vi "MatrixSwitch.vi"(8 "error in (no error)":errorcluster, 10 "Action":T1(ring), 11 "Pickering in":refnum<class "Pickering.lvclass">) -> (0 "error out":errorcluster, 2 "Continue?":bool, 3 "Pickering out":refnum<class "Pickering.lvclass">)   [LabVIEW 2013, in "Pickering.lvclass"]
uses:
  Pickering.lvclass
  InstrumentSetup.vi
  InstrControl.lvclass
panel:
  out "Display Matrix":bool[][](array[boolean])
  # "Pickering Matrix Settings"
  # "X1"
  # "X2"
  # "X3"
  # "X4"
  # "X5"
  # "X6"
  # "X7"
  # "X8"
  # "X9"
  # "X10"
  # "X11"
  # "X12"
  # "Y1"
  # "Y2"
  # "Y3"
  # "Y4"
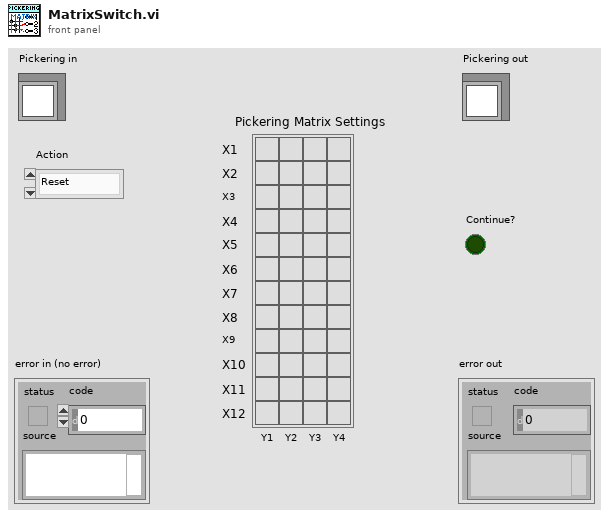
[diagram p1: front panel]
types:
  T1 = enum16{"Reset", "Ground", "Striptest SMU", "Striptest LCR", "IV", "CV", "Interstrip Cap", "Interstrip Res"}
  T2 = cluster{"Matrix address":string, "Mux1 address":string, "Mux2 address":string, "Matrix used?":bool, "Pickering":refnum<class "Pickering.lvclass">, "Matrix X Channels":cluster{"Bias Supply / SMU LO":i32, "Bias Supply / SMU HI":i32, "CV Box LO":i32, "CV Box HI":i32, "CV Box LO IN":i32, "CV Box HI IN":i32, "Volt meter LO":i32, "Volt meter HI":i32, "Mux1 C1":i32, "Mux1 C2":i32, "Mux2 C1":i32, "Mux2 C2":i32}}
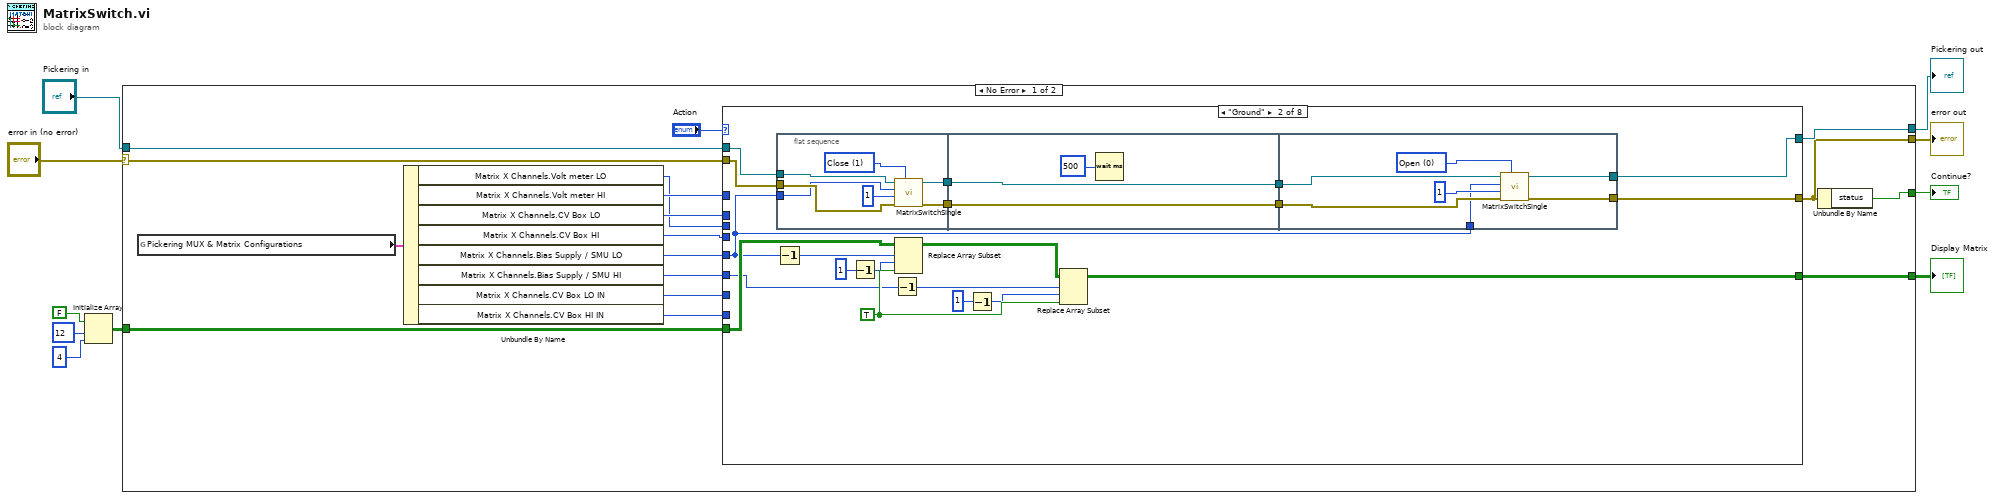
[diagram p0: block diagram]
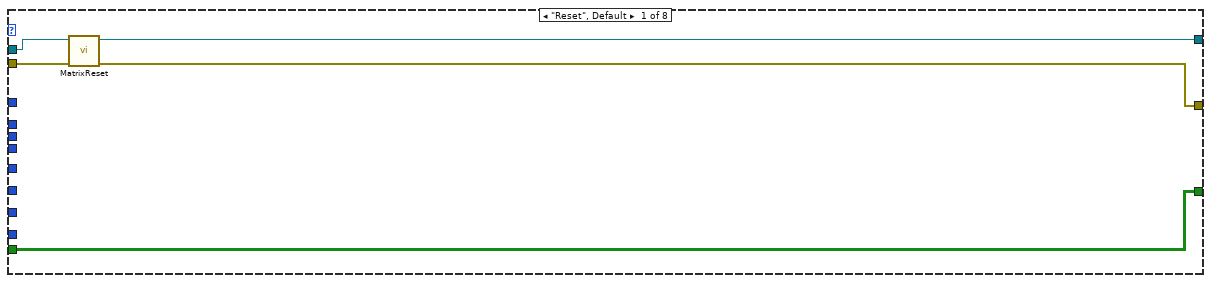
[diagram p2: hidden frame]
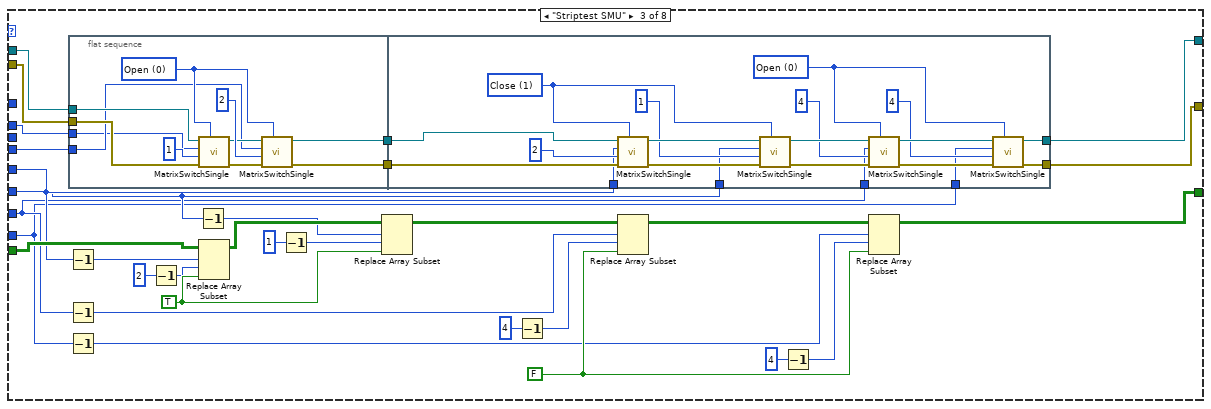
[diagram p3: hidden frame]
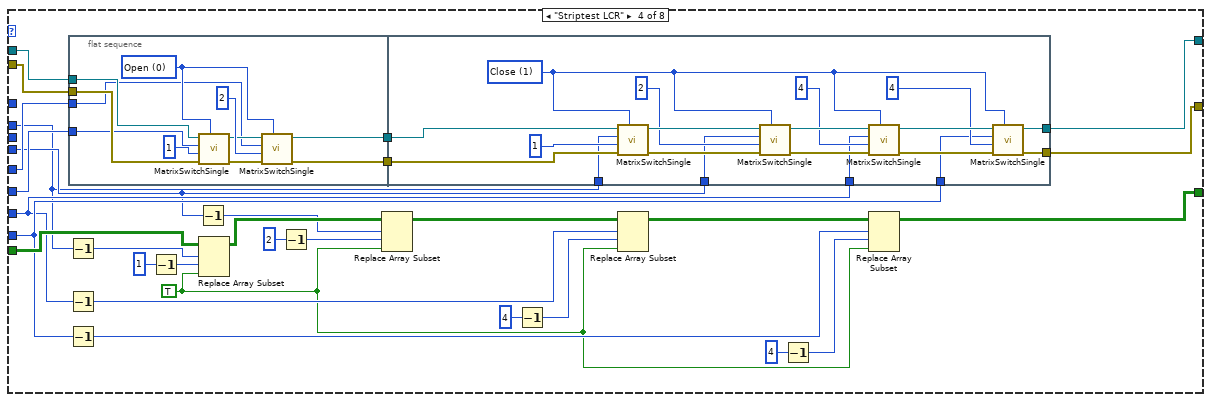
[diagram p4: hidden frame]
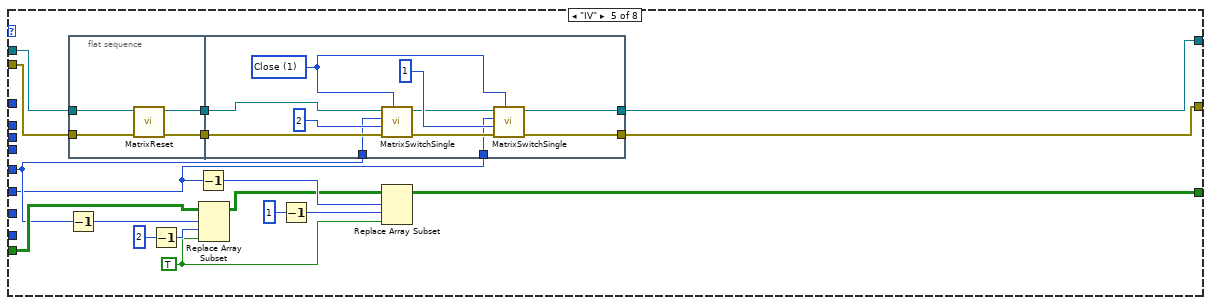
[diagram p5: hidden frame]
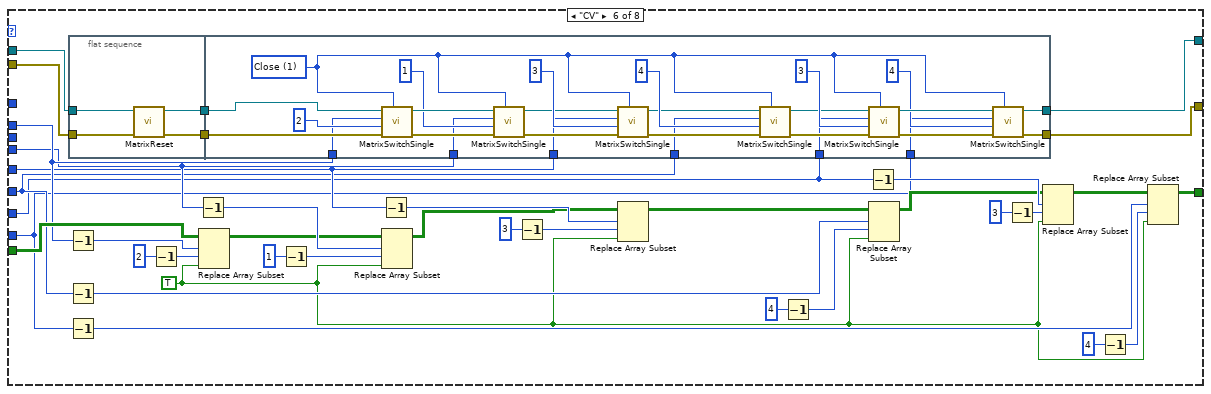
[diagram p6: hidden frame]
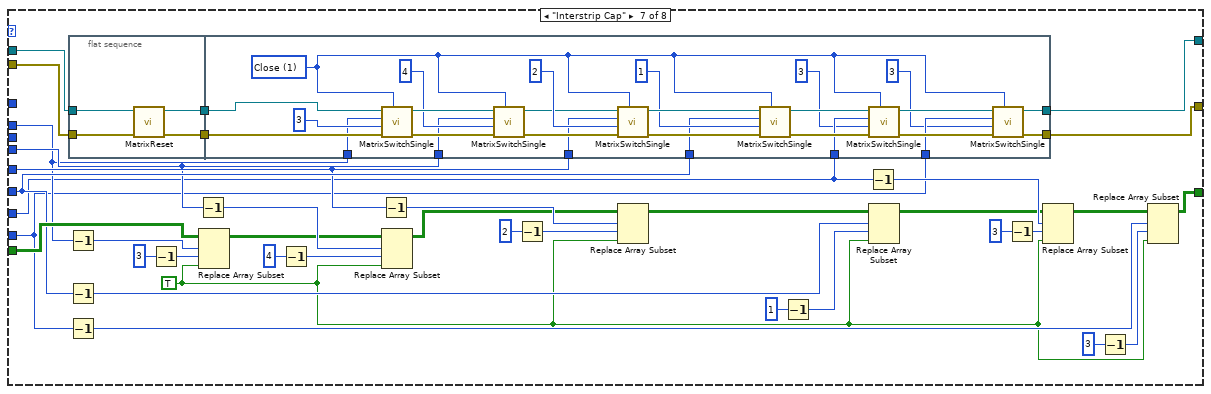
[diagram p7: hidden frame]
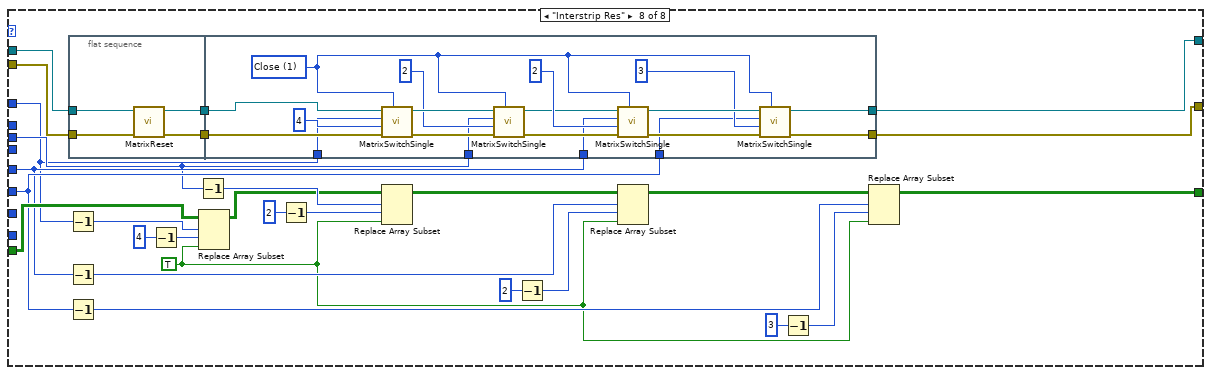
[diagram p8: hidden frame]
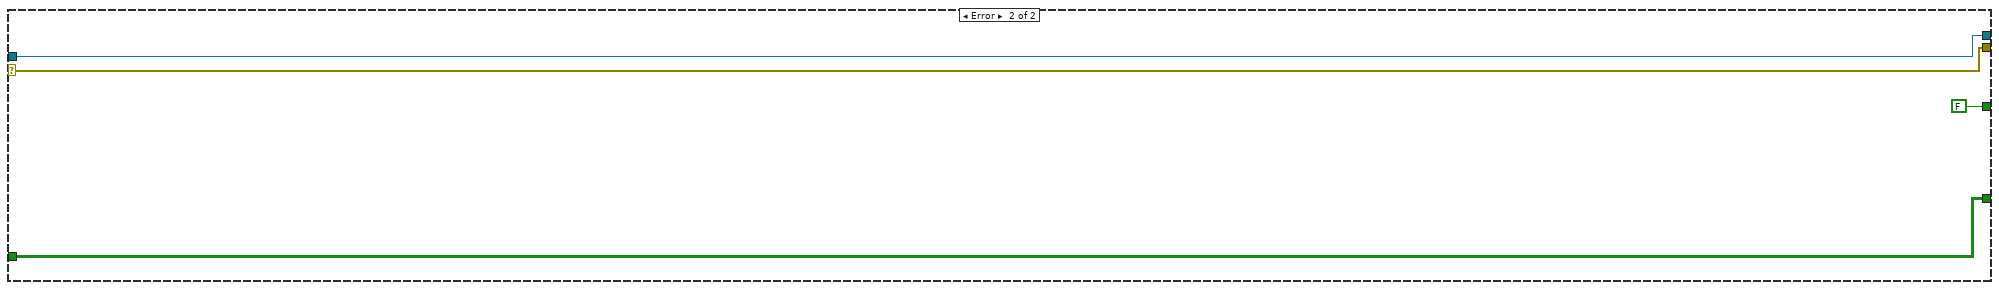
[diagram p9: hidden frame]
diagram:
  n1 = Initialize Array(FALSE, 12, 4) -> (w5:bool[][])
  n2 = case shown="No Error" "error in (no error)" {
    selector: "error in (no error)" -> [w21 w417]
    tunnel: [w24 w417] -> w2
    tunnel: [w25 w416] -> w1
    tunnel: "Pickering in" -> [w22 w416]
    tunnel: [w23 FALSE] -> w4
    tunnel: w5 -> [w27 w414]
    tunnel: [w26 w414] -> w3
    frame No Error {
      n3 = global read "InstrumentSetup.vi" "Pickering MUX & Matrix Configurations"() -> (w20:T2)
      n4 = Unbundle By Name(w20) -> ("Matrix X Channels.Volt meter LO"=w14:i32, "Matrix X Channels.Volt meter HI"=w15:i32, "Matrix X Channels.CV Box LO"=w19:i32, "Matrix X Channels.CV Box HI"=w18:i32, "Matrix X Channels.Bias Supply / SMU LO"=w12:i32, "Matrix X Channels.Bias Supply / SMU HI"=w13:i32, "Matrix X Channels.CV Box LO IN"=w17:i32, "Matrix X Channels.CV Box HI IN"=w16:i32)
      n5 = case shown="\"Ground\"" "Action" {
        tunnel: w27 -> [w32 w37 w87 w150 w200 w237 w317 w375]
        tunnel: [w32 w35 w86 w149 w201 w238 w294 w376] -> w26
        tunnel: w21 -> [w29 w52 w76 w139 w208 w236 w316 w374]
        tunnel: w22 -> [w31 w49 w78 w138 w209 w235 w315 w373]
        tunnel: [w30 w46 w81 w144 w197 w231 w311 w369] -> w25
        tunnel: [w28 w45 w80 w143 w196 w232 w312 w370] -> w24
        tunnel: w12 -> [_ w34 w73 w136 w193 w228 w308 w365]
        tunnel: w13 -> [_ w33 w72 w137 w192 w227 w309 w366]
        tunnel: w19 -> [_ _ w74 w132 _ w230 w306 _]
        tunnel: w18 -> [_ _ w75 w133 _ w229 w307 _]
        tunnel: w17 -> [_ _ w71 w134 _ w226 w298 _]
        tunnel: w16 -> [_ _ w70 w135 _ w225 w297 _]
        tunnel: w14 -> [_ _ _ _ _ _ _ w364]
        tunnel: w15 -> [_ _ _ _ _ _ _ w363]
        frame "Reset", Default {
          n6 = call-dynamic "MatrixReset.vi"("error in (no error)"=w29, "Pickering in"=w31) -> ("error out"=w28:errorcluster, "Pickering out"=w30:refnum<class "Pickering.lvclass">)  [unwired: 8 in]
        }
        frame "Ground" {
          w43 = TRUE
          n7 = Decrement(x=w34) -> (x-1=w38:i32)
          n8 = flat-sequence {
            tunnel: w52 -> [w57]
            tunnel: [w56] -> w51
            tunnel: w49 -> [w55]
            tunnel: [w54] -> w47
            tunnel: w34 -> [w53]
            tunnel: w51 -> [w61]
            tunnel: [w61] -> w50
            tunnel: [w60] -> w48
            tunnel: w47 -> [w60]
            tunnel: w50 -> [w68]
            tunnel: w48 -> [w66]
            tunnel: [w65] -> w46
            tunnel: [w64] -> w45
            tunnel: w34 -> [w63]
            frame #0 {
              w59 = u16 1 items=["Open", "Close"] ("Switch action")
              n9 = call-dynamic "MatrixSwitchSingle.vi"("Switch action"=w59, "error in (no error)"=w57, "Matrix Y"=1, "Matrix X"=w53, "Pickering in"=w55) -> ("error out"=w56:errorcluster, "Pickering out"=w54:refnum<class "Pickering.lvclass">)  [unwired: 4 in, 1 out]
            }
            frame #1 {
              n10 = Wait (ms)(milliseconds to wait=u32 500) -> ()  [unwired: 1 out]
            }
            frame #2 {
              w69 = u16 0 items=["Open", "Close"] ("Switch action")
              n11 = call-dynamic "MatrixSwitchSingle.vi"("Switch action"=w69, "error in (no error)"=w68, "Matrix Y"=1, "Matrix X"=w63, "Pickering in"=w66) -> ("error out"=w64:errorcluster, "Pickering out"=w65:refnum<class "Pickering.lvclass">)  [unwired: 4 in, 1 out]
            }
          }
          n12 = Decrement(x=1 ("Matrix Y")) -> (x-1=w39:i32)
          n13 = Decrement(x=w33) -> (x-1=w40:i32)
          n14 = Replace Array Subset(array=w37, new element=w43, index (row)=w38, index (col)=w39) -> (w44:bool[][])
          n15 = Decrement(x=1 ("Matrix Y")) -> (x-1=w41:i32)
          n16 = Replace Array Subset(array=w44, new element=w43, index (row)=w40, index (col)=w41) -> (w35:bool[][])
        }
        frame "Striptest SMU" {
          w100 = FALSE
          w99 = TRUE
          n17 = Decrement(x=w73) -> (x-1=w89:i32)
          n18 = Decrement(x=w71) -> (x-1=w94:i32)
          n19 = Decrement(x=w70) -> (x-1=w95:i32)
          n20 = flat-sequence {
            tunnel: [w107] -> w79
            tunnel: w78 -> [w105]
            tunnel: [w104] -> w77
            tunnel: w76 -> [w103]
            tunnel: w75 -> [w102]
            tunnel: w74 -> [w101]
            tunnel: [w120] -> w81
            tunnel: [w119] -> w80
            tunnel: w79 -> [w117]
            tunnel: w77 -> [w116]
            tunnel: w71 -> [w115]
            tunnel: w70 -> [w114]
            tunnel: w72 -> [w113]
            tunnel: w73 -> [w112]
            frame #0 {
              w106 = u16 0 items=["Open", "Close"] ("Switch action")
              n21 = call-dynamic "MatrixSwitchSingle.vi"("Switch action"=w106, "error in (no error)"=w103, "Matrix Y"=1, "Matrix X"=w101, "Pickering in"=w105) -> ("error out"=w110:errorcluster, "Pickering out"=w109:refnum<class "Pickering.lvclass">)  [unwired: 4 in, 1 out]
              n22 = call-dynamic "MatrixSwitchSingle.vi"("Switch action"=w106, "error in (no error)"=w110, "Matrix Y"=2, "Matrix X"=w102, "Pickering in"=w109) -> ("error out"=w107:errorcluster, "Pickering out"=w104:refnum<class "Pickering.lvclass">)  [unwired: 4 in, 1 out]
            }
            frame #1 {
              w118 = u16 0 items=["Open", "Close"] ("Switch action")
              w129 = u16 1 items=["Open", "Close"] ("Switch action")
              n23 = call-dynamic "MatrixSwitchSingle.vi"("Switch action"=w129, "error in (no error)"=w117, "Matrix Y"=2, "Matrix X"=w112, "Pickering in"=w116) -> ("error out"=w127:errorcluster, "Pickering out"=w130:refnum<class "Pickering.lvclass">)  [unwired: 4 in, 1 out]
              n24 = call-dynamic "MatrixSwitchSingle.vi"("Switch action"=w129, "error in (no error)"=w127, "Matrix Y"=1, "Matrix X"=w113, "Pickering in"=w130) -> ("error out"=w125:errorcluster, "Pickering out"=w126:refnum<class "Pickering.lvclass">)  [unwired: 4 in, 1 out]
              n25 = call-dynamic "MatrixSwitchSingle.vi"("Switch action"=w118, "error in (no error)"=w125, "Matrix Y"=4, "Matrix X"=w115, "Pickering in"=w126) -> ("error out"=w122:errorcluster, "Pickering out"=w123:refnum<class "Pickering.lvclass">)  [unwired: 4 in, 1 out]
              n26 = call-dynamic "MatrixSwitchSingle.vi"("Switch action"=w118, "error in (no error)"=w122, "Matrix Y"=4, "Matrix X"=w114, "Pickering in"=w123) -> ("error out"=w119:errorcluster, "Pickering out"=w120:refnum<class "Pickering.lvclass">)  [unwired: 4 in, 1 out]
            }
          }
          n27 = Decrement(x=2 ("Matrix Y")) -> (x-1=w88:i32)
          n28 = Decrement(x=w72) -> (x-1=w90:i32)
          n29 = Replace Array Subset(array=w87, new element=w99, index (row)=w89, index (col)=w88) -> (w92:bool[][])
          n30 = Decrement(x=1 ("Matrix Y")) -> (x-1=w91:i32)
          n31 = Replace Array Subset(array=w92, new element=w99, index (row)=w90, index (col)=w91) -> (w98:bool[][])
          n32 = Decrement(x=4 ("Matrix Y")) -> (x-1=w93:i32)
          n33 = Replace Array Subset(array=w98, new element=w100, index (row)=w94, index (col)=w93) -> (w97:bool[][])
          n34 = Decrement(x=4 ("Matrix Y")) -> (x-1=w96:i32)
          n35 = Replace Array Subset(array=w97, new element=w100, index (row)=w95, index (col)=w96) -> (w86:bool[][])
        }
        frame "Striptest LCR" {
          w142 = TRUE
          n36 = Decrement(x=w132) -> (x-1=w152:i32)
          n37 = Decrement(x=w134) -> (x-1=w157:i32)
          n38 = Decrement(x=w135) -> (x-1=w158:i32)
          n39 = flat-sequence {
            tunnel: [w168] -> w141
            tunnel: [w167] -> w140
            tunnel: w139 -> [w166]
            tunnel: w138 -> [w165]
            tunnel: w136 -> [w163]
            tunnel: w137 -> [w162]
            tunnel: [w181] -> w144
            tunnel: [w180] -> w143
            tunnel: w141 -> [w178]
            tunnel: w140 -> [w177]
            tunnel: w132 -> [w176]
            tunnel: w133 -> [w175]
            tunnel: w134 -> [w174]
            tunnel: w135 -> [w173]
            frame #0 {
              w164 = u16 0 items=["Open", "Close"] ("Switch action")
              n40 = call-dynamic "MatrixSwitchSingle.vi"("Switch action"=w164, "error in (no error)"=w166, "Matrix Y"=1, "Matrix X"=w162, "Pickering in"=w165) -> ("error out"=w171:errorcluster, "Pickering out"=w170:refnum<class "Pickering.lvclass">)  [unwired: 4 in, 1 out]
              n41 = call-dynamic "MatrixSwitchSingle.vi"("Switch action"=w164, "error in (no error)"=w171, "Matrix Y"=2, "Matrix X"=w163, "Pickering in"=w170) -> ("error out"=w167:errorcluster, "Pickering out"=w168:refnum<class "Pickering.lvclass">)  [unwired: 4 in, 1 out]
            }
            frame #1 {
              w179 = u16 1 items=["Open", "Close"] ("Switch action")
              n42 = call-dynamic "MatrixSwitchSingle.vi"("Switch action"=w179, "error in (no error)"=w177, "Matrix Y"=1, "Matrix X"=w176, "Pickering in"=w178) -> ("error out"=w188:errorcluster, "Pickering out"=w190:refnum<class "Pickering.lvclass">)  [unwired: 4 in, 1 out]
              n43 = call-dynamic "MatrixSwitchSingle.vi"("Switch action"=w179, "error in (no error)"=w188, "Matrix Y"=2, "Matrix X"=w175, "Pickering in"=w190) -> ("error out"=w186:errorcluster, "Pickering out"=w187:refnum<class "Pickering.lvclass">)  [unwired: 4 in, 1 out]
              n44 = call-dynamic "MatrixSwitchSingle.vi"("Switch action"=w179, "error in (no error)"=w186, "Matrix Y"=4, "Matrix X"=w174, "Pickering in"=w187) -> ("error out"=w183:errorcluster, "Pickering out"=w184:refnum<class "Pickering.lvclass">)  [unwired: 4 in, 1 out]
              n45 = call-dynamic "MatrixSwitchSingle.vi"("Switch action"=w179, "error in (no error)"=w183, "Matrix Y"=4, "Matrix X"=w173, "Pickering in"=w184) -> ("error out"=w180:errorcluster, "Pickering out"=w181:refnum<class "Pickering.lvclass">)  [unwired: 4 in, 1 out]
            }
          }
          n46 = Decrement(x=1 ("Matrix Y")) -> (x-1=w151:i32)
          n47 = Decrement(x=w133) -> (x-1=w153:i32)
          n48 = Replace Array Subset(array=w150, new element=w142, index (row)=w152, index (col)=w151) -> (w155:bool[][])
          n49 = Decrement(x=2 ("Matrix Y")) -> (x-1=w154:i32)
          n50 = Replace Array Subset(array=w155, new element=w142, index (row)=w153, index (col)=w154) -> (w161:bool[][])
          n51 = Decrement(x=4 ("Matrix Y")) -> (x-1=w156:i32)
          n52 = Replace Array Subset(array=w161, new element=w142, index (row)=w157, index (col)=w156) -> (w160:bool[][])
          n53 = Decrement(x=4 ("Matrix Y")) -> (x-1=w159:i32)
          n54 = Replace Array Subset(array=w160, new element=w142, index (row)=w158, index (col)=w159) -> (w149:bool[][])
        }
        frame "IV" {
          w203 = TRUE
          n55 = Decrement(x=w193) -> (x-1=w205:i32)
          n56 = flat-sequence {
            tunnel: w209 -> [w213]
            tunnel: w208 -> [w212]
            tunnel: [w211] -> w199
            tunnel: [w210] -> w198
            tunnel: w199 -> [w219]
            tunnel: w198 -> [w218]
            tunnel: [w217] -> w197
            tunnel: [w216] -> w196
            tunnel: w192 -> [w215]
            tunnel: w193 -> [w214]
            frame #0 {
              n57 = call-dynamic "MatrixReset.vi"("error in (no error)"=w212, "Pickering in"=w213) -> ("error out"=w210:errorcluster, "Pickering out"=w211:refnum<class "Pickering.lvclass">)  [unwired: 8 in]
            }
            frame #1 {
              w224 = u16 1 items=["Open", "Close"] ("Switch action")
              n58 = call-dynamic "MatrixSwitchSingle.vi"("Switch action"=w224, "error in (no error)"=w218, "Matrix Y"=2, "Matrix X"=w214, "Pickering in"=w219) -> ("error out"=w222:errorcluster, "Pickering out"=w221:refnum<class "Pickering.lvclass">)  [unwired: 4 in, 1 out]
              n59 = call-dynamic "MatrixSwitchSingle.vi"("Switch action"=w224, "error in (no error)"=w222, "Matrix Y"=1, "Matrix X"=w215, "Pickering in"=w221) -> ("error out"=w216:errorcluster, "Pickering out"=w217:refnum<class "Pickering.lvclass">)  [unwired: 4 in, 1 out]
            }
          }
          n60 = Decrement(x=2 ("Matrix Y")) -> (x-1=w204:i32)
          n61 = Decrement(x=w192) -> (x-1=w207:i32)
          n62 = Replace Array Subset(array=w200, new element=w203, index (row)=w205, index (col)=w204) -> (w202:bool[][])
          n63 = Decrement(x=1 ("Matrix Y")) -> (x-1=w206:i32)
          n64 = Replace Array Subset(array=w202, new element=w203, index (row)=w207, index (col)=w206) -> (w201:bool[][])
        }
        frame "CV" {
          w247 = TRUE
          n65 = Decrement(x=w230) -> (x-1=w260:i32)
          n66 = Decrement(x=w227) -> (x-1=w253:i32)
          n67 = Decrement(x=w225) -> (x-1=w252:i32)
          n68 = flat-sequence {
            tunnel: w236 -> [w266]
            tunnel: w235 -> [w265]
            tunnel: [w264] -> w234
            tunnel: [w263] -> w233
            tunnel: w234 -> [w276]
            tunnel: w233 -> [w275]
            tunnel: [w274] -> w232
            tunnel: [w273] -> w231
            tunnel: w230 -> [w272]
            tunnel: w229 -> [w271]
            tunnel: w228 -> [w270]
            tunnel: w227 -> [w269]
            tunnel: w226 -> [w268]
            tunnel: w225 -> [w267]
            frame #0 {
              n69 = call-dynamic "MatrixReset.vi"("error in (no error)"=w266, "Pickering in"=w265) -> ("error out"=w263:errorcluster, "Pickering out"=w264:refnum<class "Pickering.lvclass">)  [unwired: 8 in]
            }
            frame #1 {
              w279 = u16 1 items=["Open", "Close"] ("Switch action")
              n70 = call-dynamic "MatrixSwitchSingle.vi"("Switch action"=w279, "error in (no error)"=w275, "Matrix Y"=2, "Matrix X"=w272, "Pickering in"=w276) -> ("error out"=w281:errorcluster, "Pickering out"=w282:refnum<class "Pickering.lvclass">)  [unwired: 4 in, 1 out]
              n71 = call-dynamic "MatrixSwitchSingle.vi"("Switch action"=w279, "error in (no error)"=w281, "Matrix Y"=1, "Matrix X"=w271, "Pickering in"=w282) -> ("error out"=w277:errorcluster, "Pickering out"=w278:refnum<class "Pickering.lvclass">)  [unwired: 4 in, 1 out]
              n72 = call-dynamic "MatrixSwitchSingle.vi"("Switch action"=w279, "error in (no error)"=w277, "Matrix Y"=3, "Matrix X"=w270, "Pickering in"=w278) -> ("error out"=w292:errorcluster, "Pickering out"=w291:refnum<class "Pickering.lvclass">)  [unwired: 4 in, 1 out]
              n73 = call-dynamic "MatrixSwitchSingle.vi"("Switch action"=w279, "error in (no error)"=w292, "Matrix Y"=4, "Matrix X"=w269, "Pickering in"=w291) -> ("error out"=w284:errorcluster, "Pickering out"=w285:refnum<class "Pickering.lvclass">)  [unwired: 4 in, 1 out]
              n74 = call-dynamic "MatrixSwitchSingle.vi"("Switch action"=w279, "error in (no error)"=w284, "Matrix Y"=3, "Matrix X"=w268, "Pickering in"=w285) -> ("error out"=w287:errorcluster, "Pickering out"=w288:refnum<class "Pickering.lvclass">)  [unwired: 4 in, 1 out]
              n75 = call-dynamic "MatrixSwitchSingle.vi"("Switch action"=w279, "error in (no error)"=w287, "Matrix Y"=4, "Matrix X"=w267, "Pickering in"=w288) -> ("error out"=w274:errorcluster, "Pickering out"=w273:refnum<class "Pickering.lvclass">)  [unwired: 4 in, 1 out]
            }
          }
          n76 = Decrement(x=2 ("Matrix Y")) -> (x-1=w259:i32)
          n77 = Decrement(x=w229) -> (x-1=w262:i32)
          n78 = Replace Array Subset(array=w237, new element=w247, index (row)=w260, index (col)=w259) -> (w258:bool[][])
          n79 = Decrement(x=1 ("Matrix Y")) -> (x-1=w261:i32)
          n80 = Decrement(x=w228) -> (x-1=w255:i32)
          n81 = Replace Array Subset(array=w258, new element=w247, index (row)=w262, index (col)=w261) -> (w240:bool[][])
          n82 = Decrement(x=3 ("Matrix Y")) -> (x-1=w256:i32)
          n83 = Replace Array Subset(array=w240, new element=w247, index (row)=w255, index (col)=w256) -> (w257:bool[][])
          n84 = Decrement(x=4 ("Matrix Y")) -> (x-1=w254:i32)
          n85 = Decrement(x=w226) -> (x-1=w250:i32)
          n86 = Replace Array Subset(array=w257, new element=w247, index (row)=w253, index (col)=w254) -> (w239:bool[][])
          n87 = Decrement(x=3 ("Matrix Y")) -> (x-1=w249:i32)
          n88 = Replace Array Subset(array=w239, new element=w247, index (row)=w250, index (col)=w249) -> (w248:bool[][])
          n89 = Decrement(x=4 ("Matrix Y")) -> (x-1=w251:i32)
          n90 = Replace Array Subset(array=w248, new element=w247, index (row)=w252, index (col)=w251) -> (w238:bool[][])
        }
        frame "Interstrip Cap" {
          w299 = TRUE
          n91 = Decrement(x=w306) -> (x-1=w329:i32)
          n92 = Decrement(x=w309) -> (x-1=w326:i32)
          n93 = Decrement(x=w297) -> (x-1=w305:i32)
          n94 = flat-sequence {
            tunnel: w316 -> [w335]
            tunnel: w315 -> [w334]
            tunnel: [w333] -> w314
            tunnel: [w332] -> w313
            tunnel: w314 -> [w354]
            tunnel: w313 -> [w353]
            tunnel: [w338] -> w312
            tunnel: [w337] -> w311
            tunnel: w306 -> [w350]
            tunnel: w307 -> [w349]
            tunnel: w308 -> [w348]
            tunnel: w309 -> [w347]
            tunnel: w298 -> [w342]
            tunnel: w297 -> [w341]
            frame #0 {
              n95 = call-dynamic "MatrixReset.vi"("error in (no error)"=w335, "Pickering in"=w334) -> ("error out"=w332:errorcluster, "Pickering out"=w333:refnum<class "Pickering.lvclass">)  [unwired: 8 in]
            }
            frame #1 {
              w336 = u16 1 items=["Open", "Close"] ("Switch action")
              n96 = call-dynamic "MatrixSwitchSingle.vi"("Switch action"=w336, "error in (no error)"=w353, "Matrix Y"=3, "Matrix X"=w350, "Pickering in"=w354) -> ("error out"=w356:errorcluster, "Pickering out"=w357:refnum<class "Pickering.lvclass">)  [unwired: 4 in, 1 out]
              n97 = call-dynamic "MatrixSwitchSingle.vi"("Switch action"=w336, "error in (no error)"=w356, "Matrix Y"=4, "Matrix X"=w349, "Pickering in"=w357) -> ("error out"=w351:errorcluster, "Pickering out"=w352:refnum<class "Pickering.lvclass">)  [unwired: 4 in, 1 out]
              n98 = call-dynamic "MatrixSwitchSingle.vi"("Switch action"=w336, "error in (no error)"=w351, "Matrix Y"=2, "Matrix X"=w348, "Pickering in"=w352) -> ("error out"=w360:errorcluster, "Pickering out"=w361:refnum<class "Pickering.lvclass">)  [unwired: 4 in, 1 out]
              n99 = call-dynamic "MatrixSwitchSingle.vi"("Switch action"=w336, "error in (no error)"=w360, "Matrix Y"=1, "Matrix X"=w347, "Pickering in"=w361) -> ("error out"=w344:errorcluster, "Pickering out"=w343:refnum<class "Pickering.lvclass">)  [unwired: 4 in, 1 out]
              n100 = call-dynamic "MatrixSwitchSingle.vi"("Switch action"=w336, "error in (no error)"=w344, "Matrix Y"=3, "Matrix X"=w342, "Pickering in"=w343) -> ("error out"=w346:errorcluster, "Pickering out"=w345:refnum<class "Pickering.lvclass">)  [unwired: 4 in, 1 out]
              n101 = call-dynamic "MatrixSwitchSingle.vi"("Switch action"=w336, "error in (no error)"=w346, "Matrix Y"=3, "Matrix X"=w341, "Pickering in"=w345) -> ("error out"=w338:errorcluster, "Pickering out"=w337:refnum<class "Pickering.lvclass">)  [unwired: 4 in, 1 out]
            }
          }
          n102 = Decrement(x=3 ("Matrix Y")) -> (x-1=w328:i32)
          n103 = Decrement(x=w307) -> (x-1=w331:i32)
          n104 = Replace Array Subset(array=w317, new element=w299, index (row)=w329, index (col)=w328) -> (w327:bool[][])
          n105 = Decrement(x=4 ("Matrix Y")) -> (x-1=w330:i32)
          n106 = Decrement(x=w308) -> (x-1=w324:i32)
          n107 = Replace Array Subset(array=w327, new element=w299, index (row)=w331, index (col)=w330) -> (w310:bool[][])
          n108 = Decrement(x=2 ("Matrix Y")) -> (x-1=w323:i32)
          n109 = Replace Array Subset(array=w310, new element=w299, index (row)=w324, index (col)=w323) -> (w322:bool[][])
          n110 = Decrement(x=1 ("Matrix Y")) -> (x-1=w325:i32)
          n111 = Decrement(x=w298) -> (x-1=w303:i32)
          n112 = Replace Array Subset(array=w322, new element=w299, index (row)=w326, index (col)=w325) -> (w301:bool[][])
          n113 = Decrement(x=3 ("Matrix Y")) -> (x-1=w302:i32)
          n114 = Replace Array Subset(array=w301, new element=w299, index (row)=w303, index (col)=w302) -> (w300:bool[][])
          n115 = Decrement(x=3 ("Matrix Y")) -> (x-1=w304:i32)
          n116 = Replace Array Subset(array=w300, new element=w299, index (row)=w305, index (col)=w304) -> (w294:bool[][])
        }
        frame "Interstrip Res" {
          w367 = TRUE
          n117 = Decrement(x=w363) -> (x-1=w388:i32)
          n118 = Decrement(x=w365) -> (x-1=w383:i32)
          n119 = Decrement(x=w366) -> (x-1=w385:i32)
          n120 = flat-sequence {
            tunnel: w374 -> [w394]
            tunnel: w373 -> [w393]
            tunnel: [w392] -> w372
            tunnel: [w391] -> w371
            tunnel: w372 -> [w404]
            tunnel: w371 -> [w403]
            tunnel: [w402] -> w370
            tunnel: [w401] -> w369
            tunnel: w365 -> [w398]
            tunnel: w366 -> [w397]
            tunnel: w364 -> [w396]
            tunnel: w363 -> [w395]
            frame #0 {
              n121 = call-dynamic "MatrixReset.vi"("error in (no error)"=w394, "Pickering in"=w393) -> ("error out"=w391:errorcluster, "Pickering out"=w392:refnum<class "Pickering.lvclass">)  [unwired: 8 in]
            }
            frame #1 {
              w405 = u16 1 items=["Open", "Close"] ("Switch action")
              n122 = call-dynamic "MatrixSwitchSingle.vi"("Switch action"=w405, "error in (no error)"=w403, "Matrix Y"=4, "Matrix X"=w395, "Pickering in"=w404) -> ("error out"=w407:errorcluster, "Pickering out"=w408:refnum<class "Pickering.lvclass">)  [unwired: 4 in, 1 out]
              n123 = call-dynamic "MatrixSwitchSingle.vi"("Switch action"=w405, "error in (no error)"=w407, "Matrix Y"=2, "Matrix X"=w396, "Pickering in"=w408) -> ("error out"=w399:errorcluster, "Pickering out"=w400:refnum<class "Pickering.lvclass">)  [unwired: 4 in, 1 out]
              n124 = call-dynamic "MatrixSwitchSingle.vi"("Switch action"=w405, "error in (no error)"=w399, "Matrix Y"=2, "Matrix X"=w398, "Pickering in"=w400) -> ("error out"=w411:errorcluster, "Pickering out"=w412:refnum<class "Pickering.lvclass">)  [unwired: 4 in, 1 out]
              n125 = call-dynamic "MatrixSwitchSingle.vi"("Switch action"=w405, "error in (no error)"=w411, "Matrix Y"=3, "Matrix X"=w397, "Pickering in"=w412) -> ("error out"=w402:errorcluster, "Pickering out"=w401:refnum<class "Pickering.lvclass">)  [unwired: 4 in, 1 out]
            }
          }
          n126 = Decrement(x=4 ("Matrix Y")) -> (x-1=w387:i32)
          n127 = Decrement(x=w364) -> (x-1=w390:i32)
          n128 = Replace Array Subset(array=w375, new element=w367, index (row)=w388, index (col)=w387) -> (w386:bool[][])
          n129 = Decrement(x=2 ("Matrix Y")) -> (x-1=w389:i32)
          n130 = Replace Array Subset(array=w386, new element=w367, index (row)=w390, index (col)=w389) -> (w368:bool[][])
          n131 = Decrement(x=2 ("Matrix Y")) -> (x-1=w382:i32)
          n132 = Replace Array Subset(array=w368, new element=w367, index (row)=w383, index (col)=w382) -> (w381:bool[][])
          n133 = Decrement(x=3 ("Matrix Y")) -> (x-1=w384:i32)
          n134 = Replace Array Subset(array=w381, new element=w367, index (row)=w385, index (col)=w384) -> (w376:bool[][])
        }
      }
      n135 = Unbundle By Name(w24) -> ("status"=w23:bool)
    }
    frame Error {
    }
  }
  "error out" <- w2
  "Pickering out" <- w1
  "Display Matrix" <- w3
  "Continue?" <- w4
